vi "DiscreteInputsReg.vi"(7 "Discrete Inputs":bool[](array[boolean])) -> (0 "WK_UP":bool, 1 "KEY2":bool, 2 "KEY1":bool, 3 "KEY0":bool)   [LabVIEW 2013]
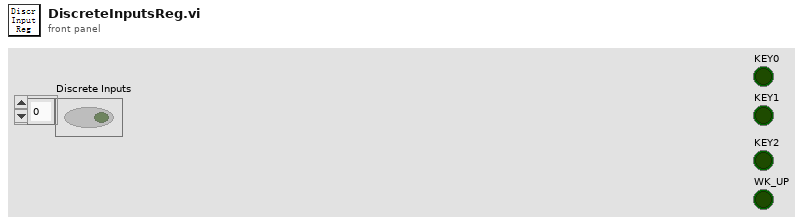
[diagram p1: front panel]
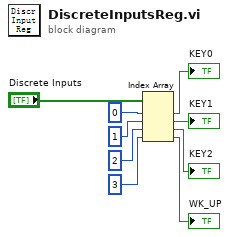
[diagram p0: block diagram]
diagram:
  n1 = Index Array(array="Discrete Inputs", index #1=0 ("索引"), index #2=1 ("索引"), index #3=2 ("索引"), index #4=3 ("索引")) -> (element #1=→"KEY0":bool, element #2=→"KEY1":bool, element #3=→"KEY2":bool, element #4=→"WK_UP":bool)
